vi "回文数与水仙花数判断(下).vi"() -> ()   [LabVIEW 2018]
panel:
  in  "下拉列表 4":u16(ring) items=["这是另一张图片", "这是一张图片", "这是一张图片"]
  in  "下拉列表 3":u16(ring)
  in  "枚举":enum16{""}(ring)
  in  "下拉列表 2":u16(ring) items=["我要自学网", "51zxw"]
  out "数值 2":dbl
  in  "下拉列表":u16(ring) items=["51自学网"=0, "我要自学网"=1, "51zxw"=4]
  out "?":bool
  out "水仙花数判断：":string
  out "回文数判断：":string
  out "?":bool
  in  "数值":i64
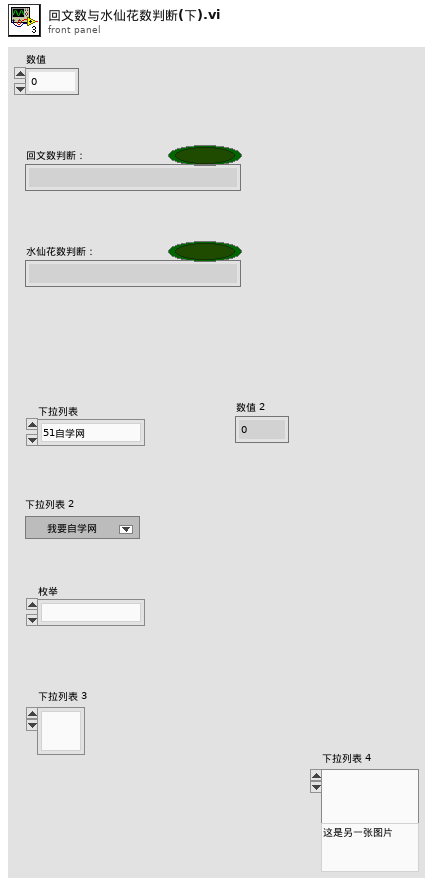
[diagram p1: front panel]
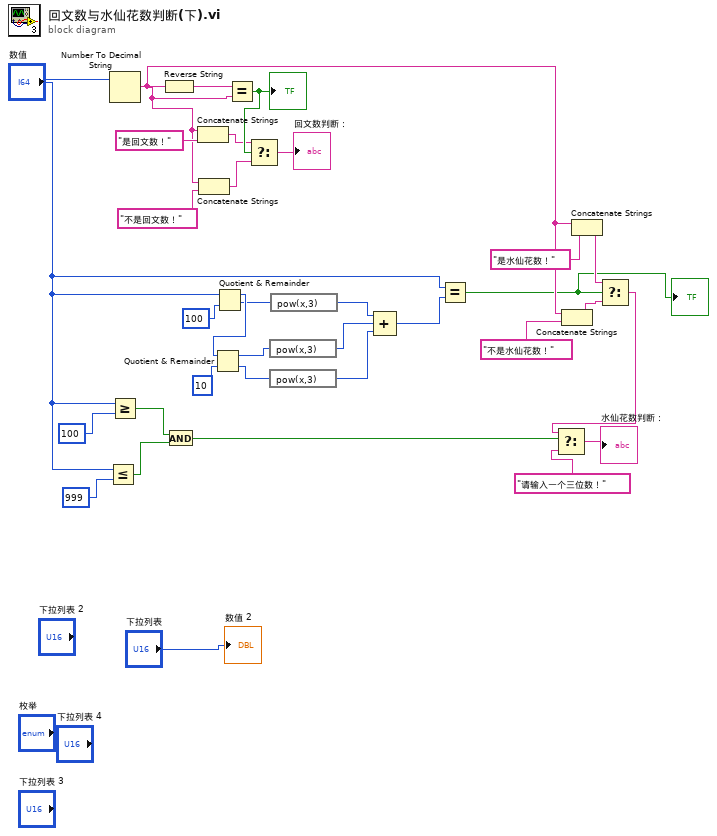
[diagram p0: block diagram]
diagram:
  n1 = Less Or Equal?(x="数值", y=999) -> (x <= y?=w24:bool)
  n2 = Number To Decimal String(number="数值") -> (decimal integer string=w5:string)  [unwired: 1 in]
  n3 = Greater Or Equal?(x="数值", y=100) -> (x >= y?=w23:bool)
  n4 = Reverse String(1:w5) -> (0:w33:string)
  n5 = And(x=w23, y=w24) -> (x .and. y?=w22:bool)
  n6 = Concatenate Strings(w5, "是回文数！") -> (w30:string)
  n7 = Concatenate Strings(w5, "不是回文数！") -> (w28:string)
  n8 = Quotient & Remainder(x="数值", y=100) -> (x-y*floor(x/y)=w17:i64, floor(x/y)=w16:i64)
  n9 = Quotient & Remainder(x=w17, y=10) -> (x-y*floor(x/y)=w15:i64, floor(x/y)=w14:i64)
  n10 = Equal?(x=w33, y=w5) -> (x = y?=w32:bool)
  "?" <- w32
  n11 = Select(t=w30, s=w32, f=w28) -> (s? t:f=→"回文数判断：":string)
  n12 = expression code="pow(x,3)"(w15) -> (w12:i64)
  n13 = expression code="pow(x,3)"(w14) -> (w13:i64)
  n14 = expression code="pow(x,3)"(w16) -> (w11:i64)
  n15 = Compound Arithmetic op=ADD(w11, w12, w13) -> (w10:i64)
  n16 = Equal?(x="数值", y=w10) -> (x = y?=w2:bool)
  "?" <- w2
  n17 = Concatenate Strings(w5, "不是水仙花数！") -> (w7:string)
  n18 = Concatenate Strings(w5, "是水仙花数！") -> (w4:string)
  n19 = Select(t=w4, s=w2, f=w7) -> (s? t:f=w3:string)
  n20 = Select(t=w3, s=w22, f="请输入一个三位数！") -> (s? t:f=→"水仙花数判断：":string)
  "数值 2" <- "下拉列表"
